vi "Reset.vi"(8 "error in":errorcluster, 11 "comport in":refnum<visa-resource-name>) -> (0 "error out":errorcluster={"status"=TRUE, "code"=-1073807339, "source"="VISA Read in FirmataClient.lvlib:Initialize.vi"}, 3 "comport out":refnum<visa-resource-name>)   [LabVIEW 2020, in "FirmataClient.lvlib"]
doc: "Builds and Sends a message according to the Firmata Protocol Requirements. \n- https://github.com/firmata/protocol\n- https://github.com/firmata/protocol/blob/master/protocol.md"
uses:
  FirmataClient.lvlib
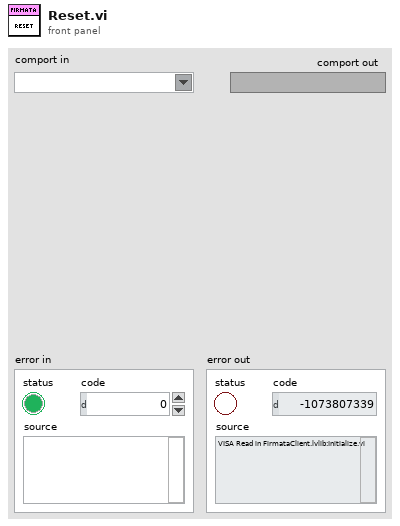
[diagram p1: front panel]
types:
  T1 = typedef "FirmataClient.lvlib/FirmataProtocolConstants.ctl" = u16
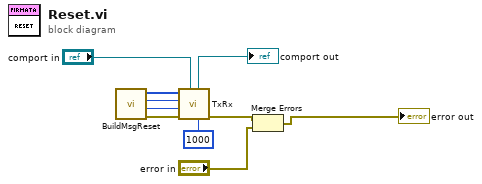
[diagram p0: block diagram]
diagram:
  n1 = call "BuildMsgReset.vi"() -> ("error out"=w8:errorcluster, "ReplyLength"=w6:i32, "ReplyFirstByte"=w5:T1, "ResetMessage"=w4:u8[])  [unwired: 8 in]
  n2 = call "TxRx.vi"("Timeout"=u32 1000, "comport in"="comport in", "error in"=w8, "Expected Reply Length"=w6, "ReplyFirstByte"=w5, "MessageToSend"=w4) -> ("error out"=w3:errorcluster, "comport out"=→"comport out":refnum<visa-resource-name>)  [unwired: 1 in, 3 out]
  n3 = Merge Errors(w3, "error in") -> (→"error out":errorcluster)
